vi "Config Measure Period.vi"(0 "VISA resource name":refnum<visa-resource-name>, 1 "Element (1: Element 1)":u16(ring)=1 items=["", "Element 1", "Element 2", "Element 3", "Element 4"], 2 "Synchronize Source (1: 1)":u16(ring)=1 items=["", "1", "2", "3", "4", "5", "6", "7", "8", "Ext"], 5 "Period Mode (0: Zero Cross)":u16(ring) items=["Zero Cross", "Cursor", "Ext Trigger"], 7 "Pattern (F: LOW)":bool, 11 "error in (no error)":errorcluster, 12 "From (0)":dbl min=0.0 max=99999.9999 format="%.4f", 13 "To (0)":dbl min=0.0 max=99999.9999 format="%.4f") -> (4 "VISA resource name out":refnum<visa-resource-name>, 15 "error out":errorcluster)   [LabVIEW 2014, in "Yokogawa.lvlib" / "Yokogawa PZ4000.lvlib"]
doc: "This VI sends the Measure Period group command to the PZ4000 series."
uses:
  Yokogawa PZ4000.lvlib
panel:
  # "HIGH"
  # "LOW"
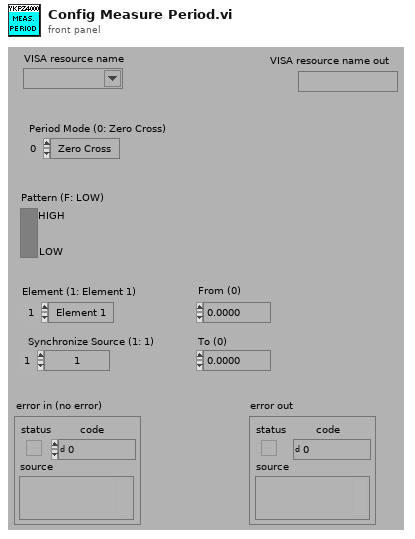
[diagram p1: front panel]
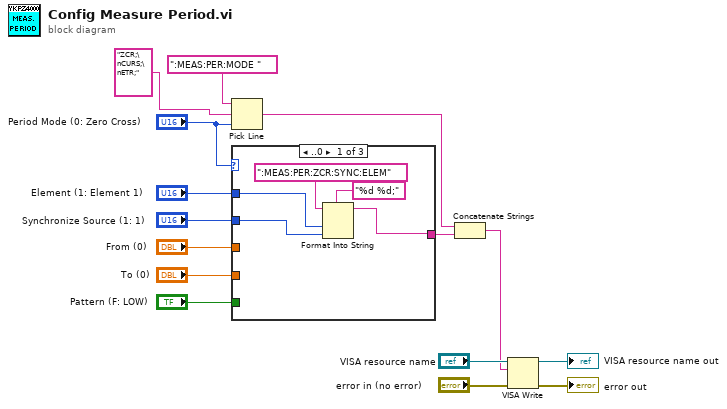
[diagram p0: block diagram]
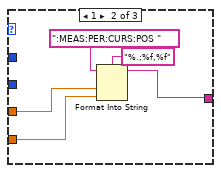
[diagram p2: hidden frame]
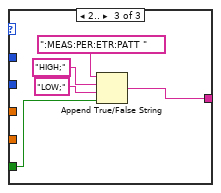
[diagram p3: hidden frame]
diagram:
  n1 = Pick Line(string ("")=":MEAS:PER:MODE ", multi-line string="ZCR;\nCURS;\nETR;", line index="Period Mode (0: Zero Cross)") -> (output string=w3:string)
  n2 = case shown="..0" "Period Mode (0: Zero Cross)" {
    tunnel: "Element (1: Element 1)" -> [w17 _ _]
    tunnel: "Synchronize Source (1: 1)" -> [w16 _ _]
    tunnel: "From (0)" -> [_ w25 _]
    tunnel: "To (0)" -> [_ w24 _]
    tunnel: "Pattern (F: LOW)" -> [_ _ w30]
    tunnel: [w18 w21 w28] -> w1
    frame ..0 {
      n3 = Format Into String(format string="%d %d;", initial string=":MEAS:PER:ZCR:SYNC:ELEM", w17, w16) -> (resulting string=w18:string)  [unwired: 1 in, 1 out]
    }
    frame 1 {
      n4 = Format Into String(format string="%.;%f,%f", initial string=":MEAS:PER:CURS:POS ", w25, w24) -> (resulting string=w21:string)  [unwired: 1 in, 1 out]
    }
    frame 2.. {
      n5 = Append True/False String(1:w30, 2:"LOW;", 3:"HIGH;", 4:":MEAS:PER:ETR:PATT ") -> (0:w28:string)
    }
  }
  n6 = Concatenate Strings(w3, w1) -> (w2:string)
  n7 = VISA Write(VISA resource name="VISA resource name", write buffer=w2, error in (no error)="error in (no error)") -> (VISA resource name out=→"VISA resource name out":refnum<visa-resource-name>, error out=→"error out":errorcluster)  [unwired: 1 out]
